vi "Tutorial 2.vi"() -> ()   [LabVIEW 2022 SP3]
panel:
  out "String":string
  in  "lastname":string
  in  "firstname":string
  in  "function name":string
  in  "Python version":string
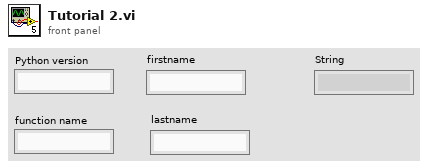
[diagram p1: front panel]
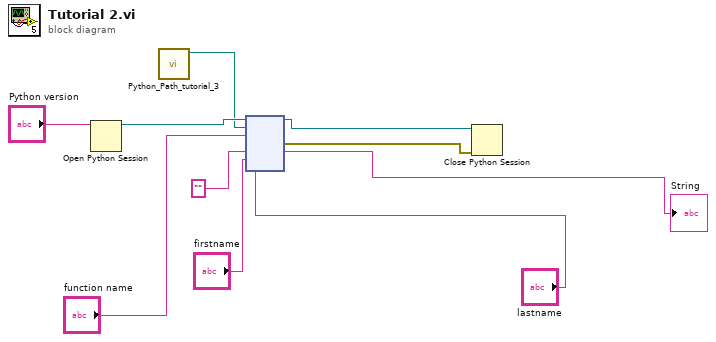
[diagram p0: block diagram]
diagram:
  n1 = Open Python Session(python version="Python version") -> (session out=w10:refnum<k35>)  [unwired: 2 in, 1 out]
  n2 = call "Python_Path_tutorial_3.vi"() -> ("appended path"=w7:path)  [unwired: 11 in]
  n3 = node(w10, w7, "function name", "", "firstname", "lastname") -> (w9:refnum<k35>, w2:errorcluster, →"String":string)  [unwired: 3 in, 2 out]
  n4 = Close Python Session(session in=w9, error in=w2) -> ()  [unwired: 1 out]
